vi "Get Elements Enum.vi"(2 "Enum Ctr":refnum<vi>) -> (0 "Enum Elements":T1[](array[typedef]))   [LabVIEW 2016]
doc: "This Vi creates an array containing all the elements in the input Enum ctrl"
uses:
  Controls/Type of Neuron.ctl
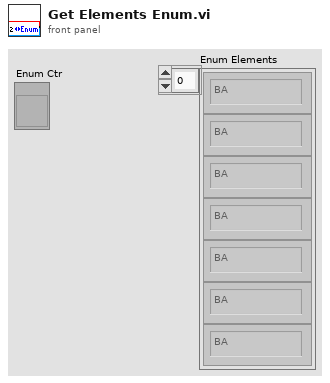
[diagram p1: front panel]
types:
  T1 = typedef "Type of Neuron.ctl" = enum16{"MF", "BA", "GO", "GC", "PC", "LU", "Glia (Dummy)"}
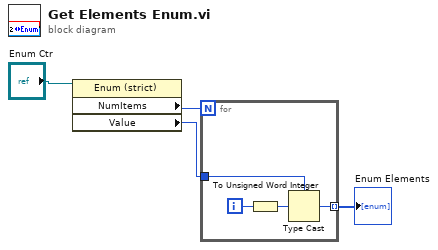
[diagram p0: block diagram]
diagram:
  n1 = property class="Enum (strict)"(reference="Enum Ctr") -> ("NumItems"=w4:u32, "Value"=w2:T1)  [unwired: 1 in, 2 out]
  n2 = for {
    N: w4 -> [_]
    tunnel: w2 -> [w7]
    tunnel: [w6] -> w3 mode=indexing
    i -> [w8]
    n3 = To Unsigned Word Integer(number=w8) -> (unsigned 16bit integer=w5:u16)
    n4 = Type Cast(type=w7, x=w5) -> (*(type *) &x=w6:T1)
  }
  "Enum Elements" <- w3
